vi "Untitled 2.vi"() -> ()   [LabVIEW 2009]
uses:
  <vilib>/Instr/_visa.llb/VISA Configure Serial Port (Instr).vi
panel:
  in  "baud rate (9600)":u32=9600
  in  "VISA resource name":refnum<visa-resource-name>
  out "decimal integer string":string
  in  "stop":bool
  out "number":u32
  in  "Cluster":cluster{"RED":bool, "BLUE":bool, "WAX":bool}
  in  "WAX OFF":dbl[](array[numeric])
  in  "WAX ON":dbl[](array[numeric])
  in  "OFF BLUE":dbl[](array[numeric])=[1000.0, 1000.0, 1000.0, 1000.0, 1000.0]
  in  "ON BLUE":dbl[](array[numeric])=[2000.0, 2000.0, 2000.0, 2000.0, 2000.0]
  in  "OFF RED":dbl[](array[numeric])=[1000.0, 2000.0, 3000.0, 4000.0, 5000.0]
  in  "ON RED":dbl[](array[numeric])=[2000.0, 1000.0, 5000.0, 3000.0, 6000.0]
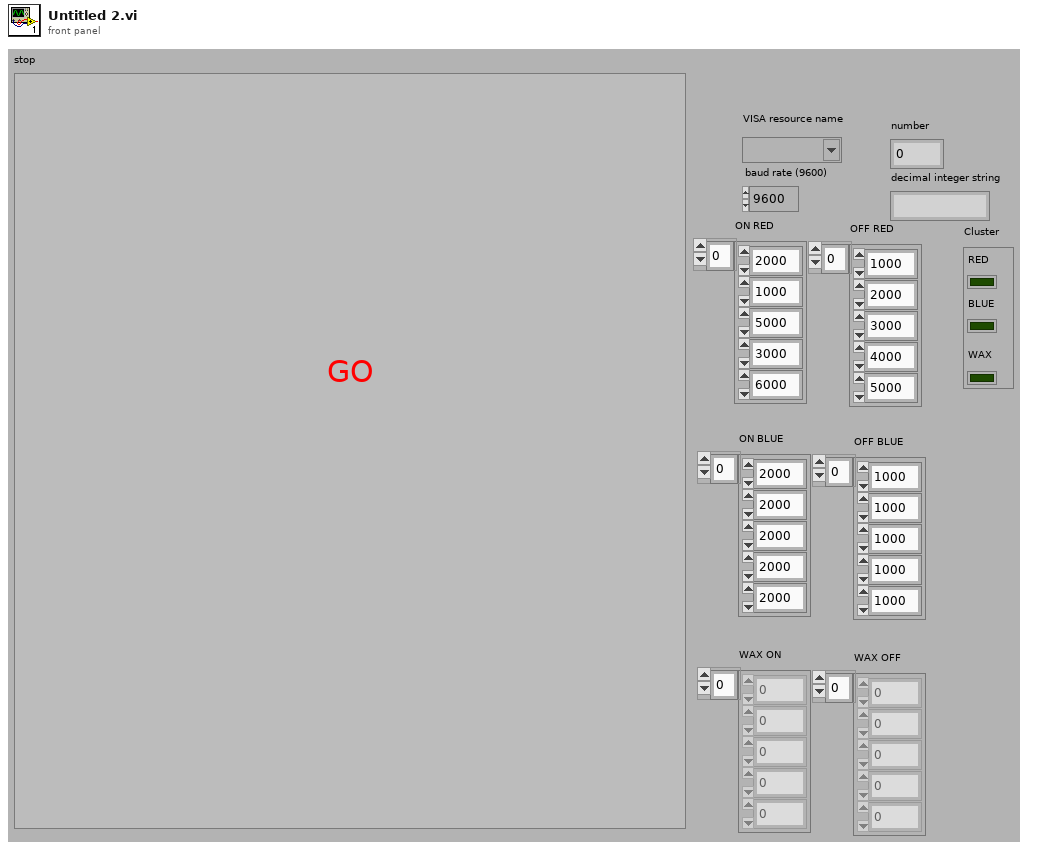
[diagram p1: front panel]
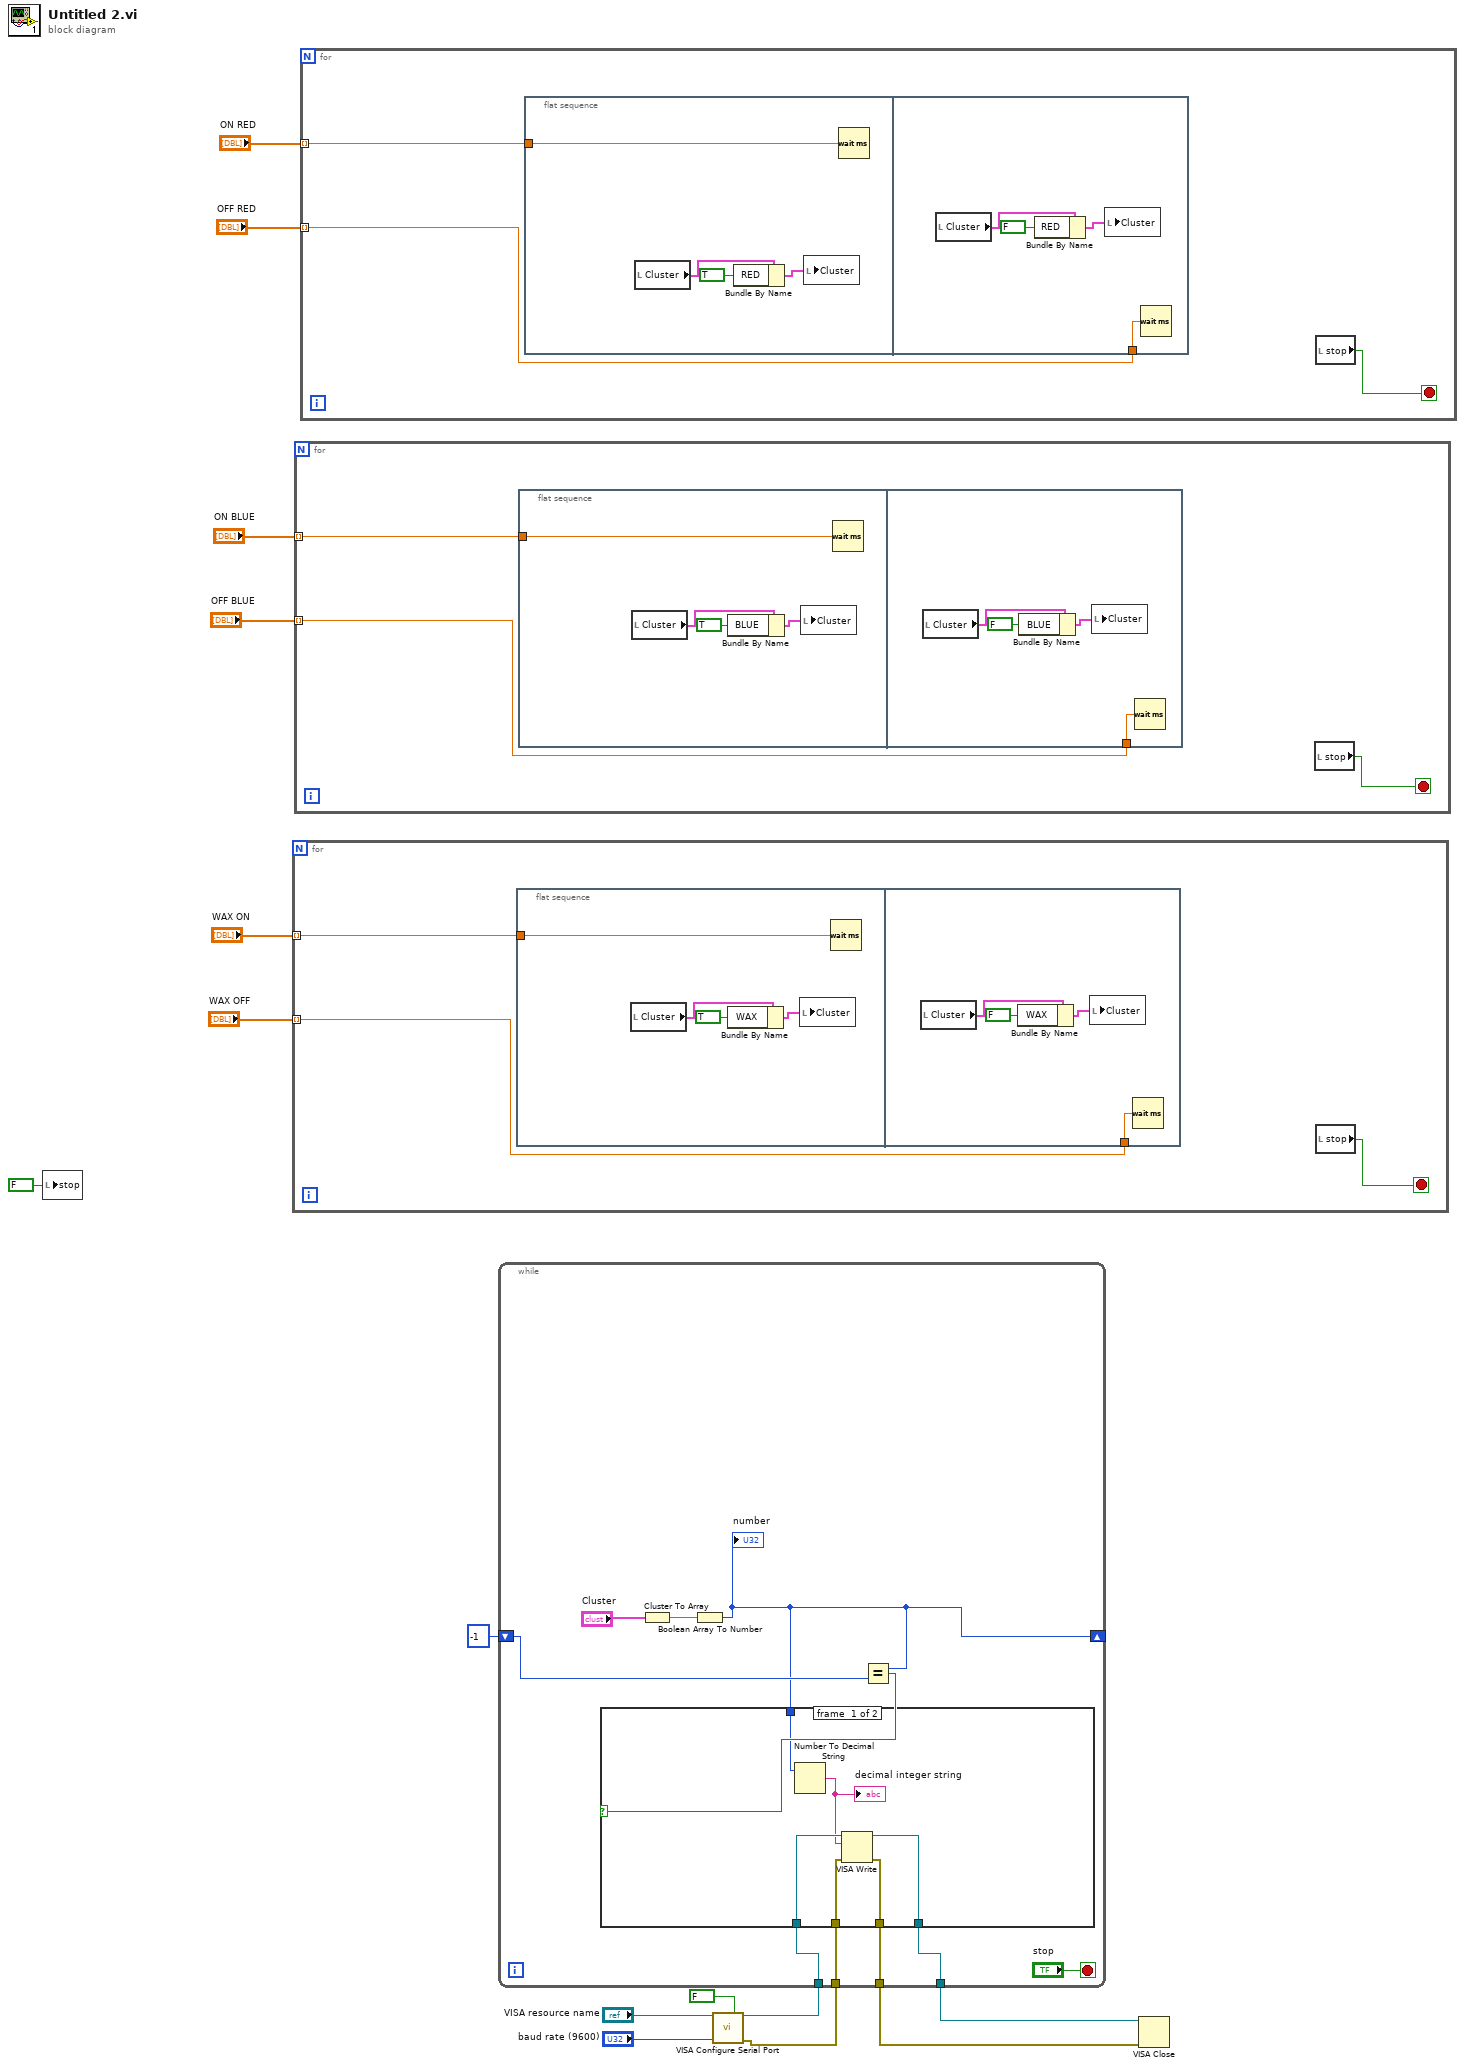
[diagram p0: block diagram]
diagram:
  n1 = local write "stop"(FALSE ("stop")) -> ()
  n2 = for {
    tunnel: "WAX ON" -> [w18] mode=indexing
    tunnel: "WAX OFF" -> [w17] mode=indexing
    stop <- w16 stop-if-true
    n3 = flat-sequence {
      tunnel: w18 -> [w22]
      tunnel: w17 -> [w26]
      frame #0 {
        n4 = local read "Cluster"() -> (w21:cluster{"RED":bool, "BLUE":bool, "WAX":bool})
        n5 = Bundle By Name(cluster=w21, "WAX"=TRUE ("RED")) -> (w19:cluster{"RED":bool, "BLUE":bool, "WAX":bool})
        n6 = local write "Cluster"(w19) -> ()
        n7 = Wait (ms)(milliseconds to wait=w22) -> ()  [unwired: 1 out]
      }
      frame #1 {
        n8 = local read "Cluster"() -> (w23:cluster{"RED":bool, "BLUE":bool, "WAX":bool})
        n9 = Bundle By Name(cluster=w23, "WAX"=FALSE ("RED")) -> (w25:cluster{"RED":bool, "BLUE":bool, "WAX":bool})
        n10 = local write "Cluster"(w25) -> ()
        n11 = Wait (ms)(milliseconds to wait=w26) -> ()  [unwired: 1 out]
      }
    }
    n12 = local read "stop"() -> (w16:bool)
  }
  n13 = for {
    tunnel: "ON BLUE" -> [w29] mode=indexing
    tunnel: "OFF BLUE" -> [w28] mode=indexing
    stop <- w27 stop-if-true
    n14 = flat-sequence {
      tunnel: w29 -> [w33]
      tunnel: w28 -> [w37]
      frame #0 {
        n15 = local read "Cluster"() -> (w30:cluster{"RED":bool, "BLUE":bool, "WAX":bool})
        n16 = Bundle By Name(cluster=w30, "BLUE"=TRUE ("RED")) -> (w32:cluster{"RED":bool, "BLUE":bool, "WAX":bool})
        n17 = local write "Cluster"(w32) -> ()
        n18 = Wait (ms)(milliseconds to wait=w33) -> ()  [unwired: 1 out]
      }
      frame #1 {
        n19 = local read "Cluster"() -> (w36:cluster{"RED":bool, "BLUE":bool, "WAX":bool})
        n20 = Bundle By Name(cluster=w36, "BLUE"=FALSE ("RED")) -> (w34:cluster{"RED":bool, "BLUE":bool, "WAX":bool})
        n21 = local write "Cluster"(w34) -> ()
        n22 = Wait (ms)(milliseconds to wait=w37) -> ()  [unwired: 1 out]
      }
    }
    n23 = local read "stop"() -> (w27:bool)
  }
  n24 = for {
    tunnel: "ON RED" -> [w40] mode=indexing
    tunnel: "OFF RED" -> [w39] mode=indexing
    stop <- w38 stop-if-true
    n25 = flat-sequence {
      tunnel: w40 -> [w44]
      tunnel: w39 -> [w48]
      frame #0 {
        n26 = local read "Cluster"() -> (w43:cluster{"RED":bool, "BLUE":bool, "WAX":bool})
        n27 = Bundle By Name(cluster=w43, "RED"=TRUE) -> (w41:cluster{"RED":bool, "BLUE":bool, "WAX":bool})
        n28 = local write "Cluster"(w41) -> ()
        n29 = Wait (ms)(milliseconds to wait=w44) -> ()  [unwired: 1 out]
      }
      frame #1 {
        n30 = local read "Cluster"() -> (w45:cluster{"RED":bool, "BLUE":bool, "WAX":bool})
        n31 = Bundle By Name(cluster=w45, "RED"=FALSE) -> (w47:cluster{"RED":bool, "BLUE":bool, "WAX":bool})
        n32 = local write "Cluster"(w47) -> ()
        n33 = Wait (ms)(milliseconds to wait=w48) -> ()  [unwired: 1 out]
      }
    }
    n34 = local read "stop"() -> (w38:bool)
  }
  n35 = call-poly "VISA Configure Serial Port"("VISA resource name"="VISA resource name", "Enable Termination\nChar (T)"=FALSE ("Enable Termination\nChar (T)"), "baud rate (9600)"="baud rate (9600)") -> ("VISA resource name out"=w8:refnum<visa-resource-name>, "error out"=w3:errorcluster)  [unwired: 11 in]
  n36 = while {
    shift-right: [w49] -> _
    shift-left: -1 -> [w56]
    tunnel: w8 -> [w54]
    tunnel: [w53] -> w7
    tunnel: w3 -> [w51]
    tunnel: [w50] -> w2
    stop <- "stop" stop-if-true
    n37 = Cluster To Array(cluster="Cluster") -> (array=w57:bool[])
    n38 = Boolean Array To Number(Boolean array=w57) -> (number=w49:u32)
    "number" <- w49
    n39 = Equal?(x=w49, y=w56) -> (x = y?=w55:bool)
    n40 = case shown="False" w55 {
      tunnel: w54 -> [w64 w66]
      tunnel: [w63 w66] -> w53
      tunnel: w49 -> [w61 _]
      tunnel: w51 -> [w60 w65]
      tunnel: [w59 w65] -> w50
      frame #0 {
        n41 = Number To Decimal String(number=w61) -> (decimal integer string=w62:string)  [unwired: 1 in]
        "decimal integer string" <- w62
        n42 = VISA Write(VISA resource name=w64, write buffer=w62, error in (no error)=w60) -> (VISA resource name out=w63:refnum<visa-resource-name>, error out=w59:errorcluster)  [unwired: 1 out]
      }
      frame #1 {
      }
    }
  }
  n43 = VISA Close(VISA resource name=w7, error in (no error)=w2) -> ()  [unwired: 1 out]
